vi "Evaluation_area.vi"(1 "X2":sgl=inf, 2 "X1":sgl=-inf, 3 "Data":cluster{dbl[], dbl[]}) -> (0 "Area":sgl format="%0.6e")   [LabVIEW 2010]
uses:
  <vilib>/Analysis/NI_AALPro.lvlib
panel:
  out "Error":i32 caption="Fehler"
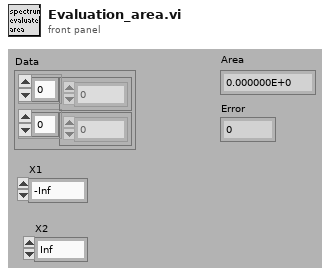
[diagram p1: front panel]
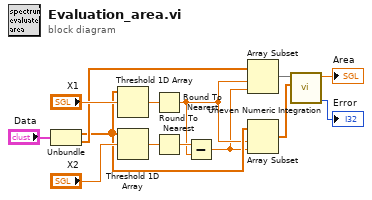
[diagram p0: block diagram]
diagram:
  n1 = Unbundle("Data") -> (w5:dbl[], w7:dbl[])
  n2 = Threshold 1D Array(2:"X1", 3:w5) -> (0:w11:dbl)  [unwired: 1 in]
  n3 = Threshold 1D Array(2:"X2", 3:w5) -> (0:w4:dbl)  [unwired: 1 in]
  n4 = Round To Nearest(number=w11) -> (nearest integer value=w2:dbl)
  n5 = Round To Nearest(number=w4) -> (nearest integer value=w3:dbl)
  n6 = Subtract(x=w3, y=w2) -> (x-y=w1:dbl)
  n7 = Array Subset(array=w7, index=w2, length=w1) -> (w8:dbl[])
  n8 = Array Subset(array=w5, index=w2, length=w1) -> (w9:dbl[])
  n9 = call <vilib>:"Uneven Numeric Integration.vi"("T"=w9, "X"=w8) -> ("error"=→"Error":i32, "result"=→"Area":dbl)  [unwired: 8 in]
